vi "FT10_Log Create TDMS File.vi"(10 "Generator Serial Number in":T1) -> (0 "t0":T2, 2 "tdms file out":T3)   [LabVIEW 2015]
doc: "Creates folder and TDMS file for data upon starting application."
uses:
  Controls/Control_Log TDMS Filename.ctl
  Controls/Control_Log t0.ctl
  Controls/Control_Serial Number.ctl
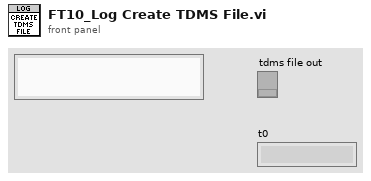
[diagram p1: front panel]
types:
  T1 = typedef "Control_Serial Number.ctl" = string
  T2 = typedef "Control_Log t0.ctl" = string
  T3 = typedef "Control_Log TDMS Filename.ctl" = refnum<k34>
  T4 = enum16{"open", "open or create", "create or replace", "create", "open (read-only)"}
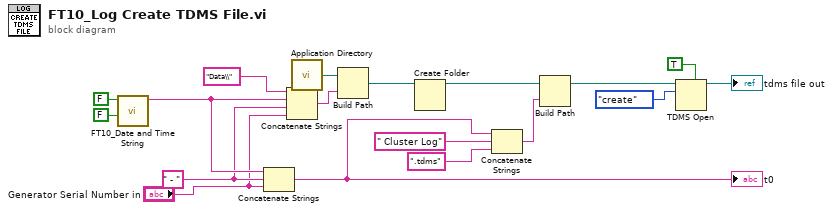
[diagram p0: block diagram]
diagram:
  w2 = " - " ("string")
  n1 = call "FT10_Date and Time String.vi"("Include msec"=FALSE, "to UTC"=FALSE) -> ("Date & Time string"=w6:string)  [unwired: 9 in]
  n2 = Concatenate Strings(w6, w2, "Generator Serial Number in") -> (w3:string)
  "t0" <- w3
  n3 = Concatenate Strings("Data\\" ("string"), w6, w2, "Generator Serial Number in") -> (w17:string)
  n4 = call <vilib>:"Application Directory.vi"() -> ("Application Directory"=w16:path)
  n5 = Build Path(base path=w16, name or relative path=w17) -> (appended path=w11:path)
  n6 = Create Folder(path (use dialog)=w11) -> (created path=w10:path)  [unwired: 2 in, 2 out]
  n7 = Concatenate Strings(w3, " Cluster Log" ("name or relative path"), ".tdms" ("string")) -> (w5:string)
  n8 = Build Path(base path=w10, name or relative path=w5) -> (appended path=w7:path)
  n9 = TDMS Open(5:TRUE ("create index file? (T)"), 10:T4."create" ("operation (0:open)"), 11:w7) -> (3:→"tdms file out":refnum<k34>)  [unwired: 4 in, 1 out]
